vi "校验信息获取.vi"(10 "料号":string, 11 "path to XML document":path caption="XML文档路径") -> (3 "校验信息":T1(array[cluster]))   [LabVIEW 2011]
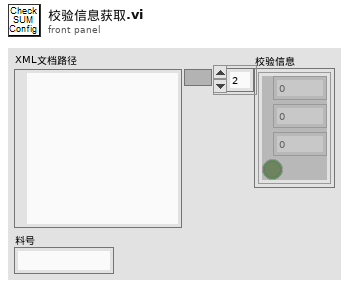
[diagram p1: front panel]
types:
  T1 = cluster{"start":i32, "length":i32, "p":i32, "H/L":bool}[]
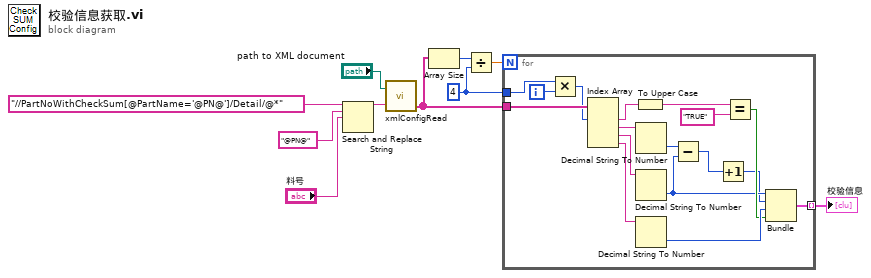
[diagram p0: block diagram]
diagram:
  w6 = 4 ("y")
  n1 = Search and Replace String(input string="//PartNoWithCheckSum[@PartName='@PN@']/Detail/@*", search string="@PN@" ("搜索字符串"), replace string="料号") -> (result string=w1:string)  [unwired: 5 in, 3 out]
  n2 = call "xmlConfigRead.vi"("path to XML document"="path to XML document", "XPath expression"=w1) -> ("OutParaArray"=w7:string[])  [unwired: 2 out]
  n3 = Array Size(array=w7) -> (size(s)=w9:i32)
  n4 = Divide(x=w9, y=w6) -> (x/y=w8:dbl)
  n5 = for {
    N: w8 -> [_]
    tunnel: w7 -> [w25]
    tunnel: w6 -> [w27]
    tunnel: [w15] -> w5 mode=indexing
    i -> [w26]
    n6 = Multiply(x=w27, y=w26) -> (x*y=w24:i32)
    n7 = Index Array(array=w25, index #1=w24) -> (element #1=w23:string, element #2=w20:string, element #3=w19:string, element #4=w18:string)  [unwired: 3 in]
    n8 = To Upper Case(1:w23) -> (0:w22:string)
    n9 = Decimal String To Number(string=w20) -> (number=w14:i32)  [unwired: 2 in, 1 out]
    n10 = Decimal String To Number(string=w19) -> (number=w13:i32)  [unwired: 2 in, 1 out]
    n11 = Decimal String To Number(string=w18) -> (number=w17:i32)  [unwired: 2 in, 1 out]
    n12 = Subtract(x=w14, y=w13) -> (x-y=w12:i32)
    n13 = Increment(x=w12) -> (x+1=w11:i32)
    n14 = Equal?(x=w22, y="TRUE") -> (x = y?=w16:bool)
    n15 = Bundle(w13, w11, w17, w16) -> (w15:cluster{i32, i32, i32, bool})  [unwired: 1 in]
  }
  "校验信息" <- w5
